vi "CAN Log Queue  FGV.vi"(6 "CAN FGV State":T1, 8 "error in":errorcluster, 10 "Current Scoket":i16, 11 "Log queue in":refnum<queue>) -> (0 "error out":errorcluster, 3 "Log queue out":refnum<queue>)   [LabVIEW 2023, in "LTT_TeststandSteptypes.lvlib"]
uses:
  LTT_TeststandSteptypes.lvlib
  Control/CAN FGV State.ctl
panel:
  out "Array":refnum<queue>[](array[refnum])
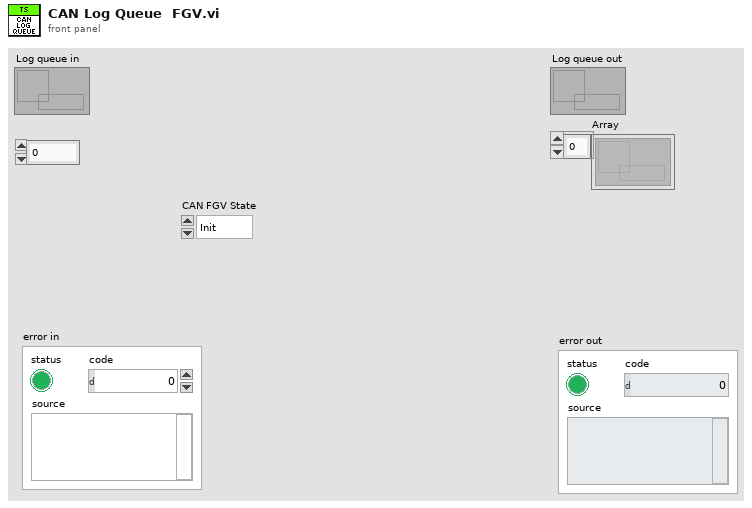
[diagram p1: front panel]
types:
  T1 = typedef "LTT_TeststandSteptypes.lvlib/CAN FGV State.ctl" = enum16{"Init", "Get", "Set"}
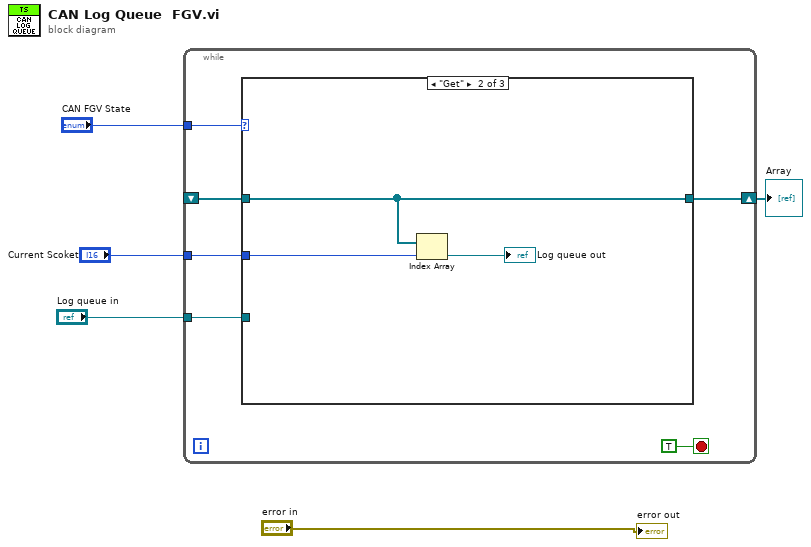
[diagram p0: block diagram]
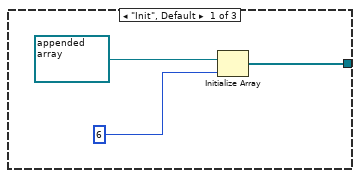
[diagram p2: hidden frame]
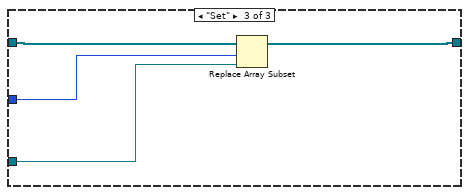
[diagram p3: hidden frame]
diagram:
  n1 = while {
    tunnel: "CAN FGV State" -> [w10]
    tunnel: "Log queue in" -> [w9]
    shift-right: [w8] -> w1
    shift-left: _ -> [w7]
    tunnel: "Current Scoket" -> [w6]
    stop <- TRUE stop-if-true
    n2 = case shown="\"Get\"" w10 {
      tunnel: w9 -> [_ _ w18]
      tunnel: [w13 w17 w20] -> w8
      tunnel: w7 -> [_ w17 w21]
      tunnel: w6 -> [_ w16 w19]
      frame "Init", Default {
        n3 = Initialize Array(refnum<queue> refnum ("queue out"), 6 ("dimension size")) -> (w13:refnum<queue>[])
      }
      frame "Get" {
        n4 = Index Array(array=w17, index=w16) -> (element=→"Log queue out":refnum<queue>)
      }
      frame "Set" {
        n5 = Replace Array Subset(array=w21, new element=w18, index=w19) -> (w20:refnum<queue>[])
      }
    }
  }
  "Array" <- w1
  "error out" <- "error in"
